vi "Find Spline Segment.vi"(1 "knots":dbl[](array[numeric]), 2 "position":dbl) -> (0 "spline segment idx":i32)   [LabVIEW 2019]
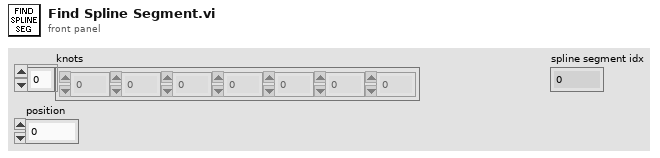
[diagram p1: front panel]
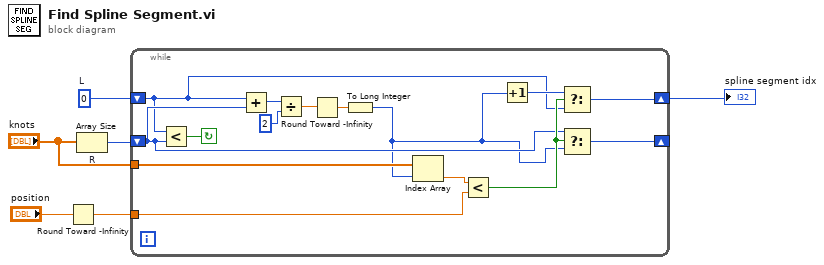
[diagram p0: block diagram]
diagram:
  w6 = 0  # L
  n1 = Round Toward -Infinity(1:"position") -> (0:w1:dbl)
  n2 = Array Size "R"(array="knots") -> (size(s)=w5:i32)
  n3 = while {
    tunnel: "knots" -> [w17]
    tunnel: w1 -> [w15]
    shift-right: [w8] -> w3
    shift-left: w6 -> [w11]
    shift-right: [w7] -> _
    shift-left: w5 -> [w13]
    stop <- w21 continue-if-true
    n4 = Less?(x=w11, y=w13) -> (x < y?=w21:bool)
    n5 = Add(x=w11, y=w13) -> (x+y=w20:i32)
    n6 = Divide(x=w20, y=2) -> (x/y=w18:dbl)
    n7 = Round Toward -Infinity(1:w18) -> (0:w10:dbl)
    n8 = To Long Integer(number=w10) -> (32bit integer=w9:i32)
    n9 = Index Array(array=w17, index=w9) -> (element=w16:dbl)
    n10 = Less?(x=w16, y=w15) -> (x < y?=w14:bool)
    n11 = Increment(x=w9) -> (x+1=w12:i32)
    n12 = Select(t=w12, s=w14, f=w11) -> (s? t:f=w8:i32)
    n13 = Select(t=w13, s=w14, f=w9) -> (s? t:f=w7:i32)
  }
  "spline segment idx" <- w3
